vi "ME_acquire_5.vi"() -> ()   [LabVIEW 2015]
doc: "Use this template to build a producer/consumer design pattern. Use this template when you need to execute a process, such as data analysis, when a data source, such as a triggered acquisition, produces data at an uneven rate and you need to execute the process when the data becomes available."
uses:
  Mode.ctl
  oxford_driver/Oxford Drivers/BUSGEN.LLB/OxfordAddress.ctl
  <vilib>/Utility/file.llb/Write Delimited Spreadsheet (DBL).vi
  <vilib>/express/express arith-compare/Formula/XNode/ExpressFormulaBlockNode.xnode
  <vilib>/gmath/NI_Gmath.lvlib
panel:
  in  "stop 2":bool
  in  "dB":dbl=0.005
  in  "Dwell Time (ms)":u32=1
  out "appended array":dbl[][](array[numeric])
  in  "Magnet":bool
  out "Actual B Field (T)":dbl
  out "Actual Temperature (K)":dbl
  out "Actual Current (pA)":dbl
  in  "Sweep Field":bool
  in  "Tab Control":T1(tab)
  out "P(T)":cluster{dbl[], dbl[]}(graph)
  out "I(T)":cluster{dbl[], dbl[]}(graph)
  in  "Set temperature (K)":dbl=4.5
  in  "Temp Ramping Rate (K/min)":dbl=10.0
  in  "Heater Range":enum16{"Off", "Low", "Medium", "High"}(ring)
  in  "Heater On/Off":bool
  out "I(B) /Averaged/":cluster{"B array":dbl[], dbl[]}[](graph)
  out "I(B) 3":cluster{dbl[], dbl[]}[](graph)
  in  "Go to Set":bool
  in  "Set Field (T)":dbl=0.3
  in  "Field To Zero":bool
  in  "Sweep Rate (T/min)":dbl=2.0 format="%.6f"
  in  "Min Field (T)":dbl
  in  "Max Field (T)":dbl
  out "Up/Down":bool
  in  "Measure Noise":bool
  in  "Cycles":i32
  in  "maximum value":dbl=10.0 format="%0.2f"
  in  "minimum value":dbl=-10.0 format="%0.2f"
  in  "physical channels":tag="Dev1/ai1"
  out "PSD (pA/Hz^1/2) Peaks Removed":cluster{"f0":dbl, "df":dbl, "magnitude":dbl[]}(graph)
  out "PSD (pA/Hz^1/2)":cluster{"f0":dbl, "df":dbl, "magnitude":dbl[]}(graph)
  out "Current (pA) Filtered":waveform(dbl)(graph)
  out "Current (pA)":dbl[](graph)
  in  "Samples per channel":i32=1000
  in  "Rate":dbl=1000.0 format="%0.2f"
  in  "Cut-Off Frequency":dbl=100.0 caption="Lower Cut-Off"
  in  "Filter On":bool
  in  "Calibrate":bool
  in  "IV converter":refnum<visa-resource-name>="GPIB0::20::INSTR"
  in  "Magnetic Field":refnum<visa-resource-name>="GPIB0::21::INSTR"
  out "Time Lag":dbl=0.0500025749206543
  in  "Lake Shore":refnum<visa-resource-name>="GPIB0::11::INSTR"
  in  "Temp Refresh (s)":dbl=1.0
  in  "Sampling rate (Hz)":dbl=10.0
  in  "Gain (V/A)":dbl=1000000000.0
  in  "Sample area (mm^2)":dbl=3.9
  out "B_V":cluster{dbl[], "Best Linear Fit":dbl[]}[](graph)=[{[-0.00854253601, 0.00626134724, 0.0219834428, 0.0379117736, 0.0535871506, 0.0694316728, 0.0851615152, 0.100816481, 0.116478038, 0.132148461, 0.147876163, 0.16341701, 0.178976744, 0.194563632, 0.210251739, 0.225738944, 0.241298253, 0.256806034, 0.272344374, 0.287933477, 0.303494709, 0.318997125, 0.334591297, 0.350146681, 0.365618053, 0.380940961, 0.39666457, 0.412213675, 0.427724671, 0.443221444, 0.458760641, 0.474360042, 0.489915118, 0.505330598, 0.520967119, 0.536347531, 0.551813711, 0.567441155, 0.582995861, 0.598507522, 0.614041988, 0.629563151, 0.645106262, 0.660611914, 0.676136149, 0.691553948, 0.7071244, 0.72262999, 0.738171137, 0.753700392, 0.76919513, 0.784778028, 0.800215944, 0.8156961, 0.831325434, 0.846852183, 0.862326812, 0.877819169, 0.893312568, 0.90888536, 0.924354789], "Best Linear Fit"=[0.0, 0.005, 0.01, 0.015, 0.02, 0.025, 0.03, 0.035, 0.04, 0.045, 0.05, 0.055, 0.06, 0.065, 0.07, 0.075, 0.08, 0.085, 0.09, 0.095, 0.1, 0.105, 0.11, 0.115, 0.12, 0.125, 0.13, 0.135, 0.14, 0.145, 0.15, 0.155, 0.16, 0.165, 0.17, 0.175, 0.18, 0.185, 0.19, 0.195, 0.2, 0.205, 0.21, 0.215, 0.22, 0.225, 0.23, 0.235, 0.24, 0.245, 0.25, 0.255, 0.26, 0.265, 0.27, 0.275, 0.28, 0.285, 0.29, 0.295, 0.3]}, {[-0.00854253601, 0.00626134724, 0.0219834428, 0.0379117736, 0.0535871506, 0.0694316728, 0.0851615152, 0.100816481, 0.116478038, 0.132148461, 0.147876163, 0.16341701, 0.178976744, 0.194563632, 0.210251739, 0.225738944, 0.241298253, 0.256806034, 0.272344374, 0.287933477, 0.303494709, 0.318997125, 0.334591297, 0.350146681, 0.365618053, 0.380940961, 0.39666457, 0.412213675, 0.427724671, 0.443221444, 0.458760641, 0.474360042, 0.489915118, 0.505330598, 0.520967119, 0.536347531, 0.551813711, 0.567441155, 0.582995861, 0.598507522, 0.614041988, 0.629563151, 0.645106262, 0.660611914, 0.676136149, 0.691553948, 0.7071244, 0.72262999, 0.738171137, 0.753700392, 0.76919513, 0.784778028, 0.800215944, 0.8156961, 0.831325434, 0.846852183, 0.862326812, 0.877819169, 0.893312568, 0.90888536, 0.924354789], "Best Linear Fit"=[-0.00022554388023060128, 0.004536267537808887, 0.009593430775915074, 0.014716931562355689, 0.01975906732634002, 0.024855610270593523, 0.029915265354287977, 0.03495083565949541, 0.03998852608757118, 0.045029068349812316, 0.05008803495326229, 0.055086897848955874, 0.060091835929837946, 0.06510550835596321, 0.07015173884687344, 0.07513334727738563, 0.08013814865293042, 0.08512637555172443, 0.0901244320467579, 0.09513881694893507, 0.10014423687592358, 0.10513073807087174, 0.11014675346564809, 0.1151502923271957, 0.12012680792099008, 0.1250555686413888, 0.1301132186920259, 0.13511473785283767, 0.14010399888730068, 0.14508868495702945, 0.1500870171143548, 0.15510471446726903, 0.16010815425765457, 0.16506669165212906, 0.17009632901003072, 0.1750435864450521, 0.18001843198211442, 0.1850451496356715, 0.19004847041199868, 0.1950379453501071, 0.20003475573578386, 0.20502728708357412, 0.21002687821664084, 0.21501442030211, 0.220007939788244, 0.2249672231113706, 0.22997560874002893, 0.23496313088260184, 0.23996209027618054, 0.24495722449359253, 0.24994125598600042, 0.2549536449902534, 0.25991939913989753, 0.2648987401917687, 0.26992606578200207, 0.2749203939204135, 0.2798979571595809, 0.2848812227804405, 0.2898648235706211, 0.2948739618827834, 0.2998498524919418]}]
  out "V_I":cluster{dbl[], "Best Linear Fit":dbl[]}[](graph)=[{[0.0, 0.035, 0.069, 0.104, 0.138, 0.173, 0.208, 0.242, 0.277, 0.311, 0.346, 0.38, 0.415, 0.45, 0.484, 0.519, 0.553, 0.588, 0.623, 0.657, 0.692, 0.726, 0.761, 0.796, 0.83, 0.865, 0.899, 0.934, 0.969, 1.003, 1.038, 1.072, 1.107, 1.141, 1.176, 1.211, 1.245, 1.28, 1.314, 1.349, 1.384, 1.418, 1.453, 1.487, 1.522, 1.557, 1.591, 1.626, 1.66, 1.695, 1.73, 1.764, 1.799, 1.833, 1.868, 1.902, 1.937, 1.972, 2.006, 2.041, 2.075], "Best Linear Fit"=[-0.00854253601, 0.00626134724, 0.0219834428, 0.0379117736, 0.0535871506, 0.0694316728, 0.0851615152, 0.100816481, 0.116478038, 0.132148461, 0.147876163, 0.16341701, 0.178976744, 0.194563632, 0.210251739, 0.225738944, 0.241298253, 0.256806034, 0.272344374, 0.287933477, 0.303494709, 0.318997125, 0.334591297, 0.350146681, 0.365618053, 0.380940961, 0.39666457, 0.412213675, 0.427724671, 0.443221444, 0.458760641, 0.474360042, 0.489915118, 0.505330598, 0.520967119, 0.536347531, 0.551813711, 0.567441155, 0.582995861, 0.598507522, 0.614041988, 0.629563151, 0.645106262, 0.660611914, 0.676136149, 0.691553948, 0.7071244, 0.72262999, 0.738171137, 0.753700392, 0.76919513, 0.784778028, 0.800215944, 0.8156961, 0.831325434, 0.846852183, 0.862326812, 0.877819169, 0.893312568, 0.90888536, 0.924354789]}, {[0.0, 0.035, 0.069, 0.104, 0.138, 0.173, 0.208, 0.242, 0.277, 0.311, 0.346, 0.38, 0.415, 0.45, 0.484, 0.519, 0.553, 0.588, 0.623, 0.657, 0.692, 0.726, 0.761, 0.796, 0.83, 0.865, 0.899, 0.934, 0.969, 1.003, 1.038, 1.072, 1.107, 1.141, 1.176, 1.211, 1.245, 1.28, 1.314, 1.349, 1.384, 1.418, 1.453, 1.487, 1.522, 1.557, 1.591, 1.626, 1.66, 1.695, 1.73, 1.764, 1.799, 1.833, 1.868, 1.902, 1.937, 1.972, 2.006, 2.041, 2.075], "Best Linear Fit"=[-0.007846580254753975, 0.007882153481927697, 0.02316149482613275, 0.03889022856281441, 0.054169569907019474, 0.06989830364370113, 0.08562703738038281, 0.10090637872458785, 0.11663511246126955, 0.1319144538054746, 0.14764318754215625, 0.1629225288863613, 0.17865126262304296, 0.19437999635972467, 0.2096593377039297, 0.22538807144061138, 0.24066741278481643, 0.25639614652149806, 0.27212488025817977, 0.2874042216023848, 0.3031329553390665, 0.31841229668327153, 0.3341410304199532, 0.3498697641566349, 0.3651491055008399, 0.3808778392375216, 0.39615718058172666, 0.4118859143184083, 0.42761464805509, 0.442893989399295, 0.45862272313597674, 0.4739020644801818, 0.48963079821686345, 0.5049101395610684, 0.5206388732977502, 0.5363676070344319, 0.5516469483786369, 0.5673756821153185, 0.5826550234595236, 0.5983837571962053, 0.6141124909328869, 0.629391832277092, 0.6451205660137737, 0.6603999073579787, 0.6761286410946604, 0.691857374831342, 0.7071367161755471, 0.7228654499122288, 0.7381447912564338, 0.7538735249931156, 0.7696022587297972, 0.7848816000740022, 0.8006103338106839, 0.815889675154889, 0.8316184088915707, 0.8468977502357756, 0.8626264839724573, 0.878355217709139, 0.893634559053344, 0.9093632927900257, 0.9246426341342309]}]
  out "B0 (T)":dbl=0.0025222449819540214
  out "B/V (T/V)":dbl=0.321659617116981
  out "I0 (A)":dbl=-0.007846580254753975
  out "V/I (Ohm)":dbl=0.44939239247661916
  in  "dt (s)":dbl=0.05
  in  "Temp/Magnetic Field":bool
  out "Save":dbl[][](array[numeric])
  out "output array":dbl[][](array[numeric])
  out "index":i8
  out "Read?":bool
  out "Magnetic Field (T)":dbl[](array[numeric])
  out "Reset":bool
  out "Measured Current (pA)":dbl[](array[numeric])
  out "Elapsed Time (s)":dbl[](array[numeric])
  out "Start time":timestamp
  in  "Enum":T2
  out "B array":dbl[](array[numeric])
  in  "dB (T)":dbl=0.0001
  in  "Counter":i8
  out "L magnet (H)":dbl
  out "R magnet (mOhm)":dbl
  out "Actual Current (R0)":dbl
  out "Actual Field (T)":dbl
  out "Temperature array":dbl[](array[numeric])
  in  "New Measurement File":bool
  out "Measurement File":path
  out "refnum out":refnum<file>
  in  "Measuring":bool
  in  "Measure (Start/Pause)":bool
  in  "stop":bool
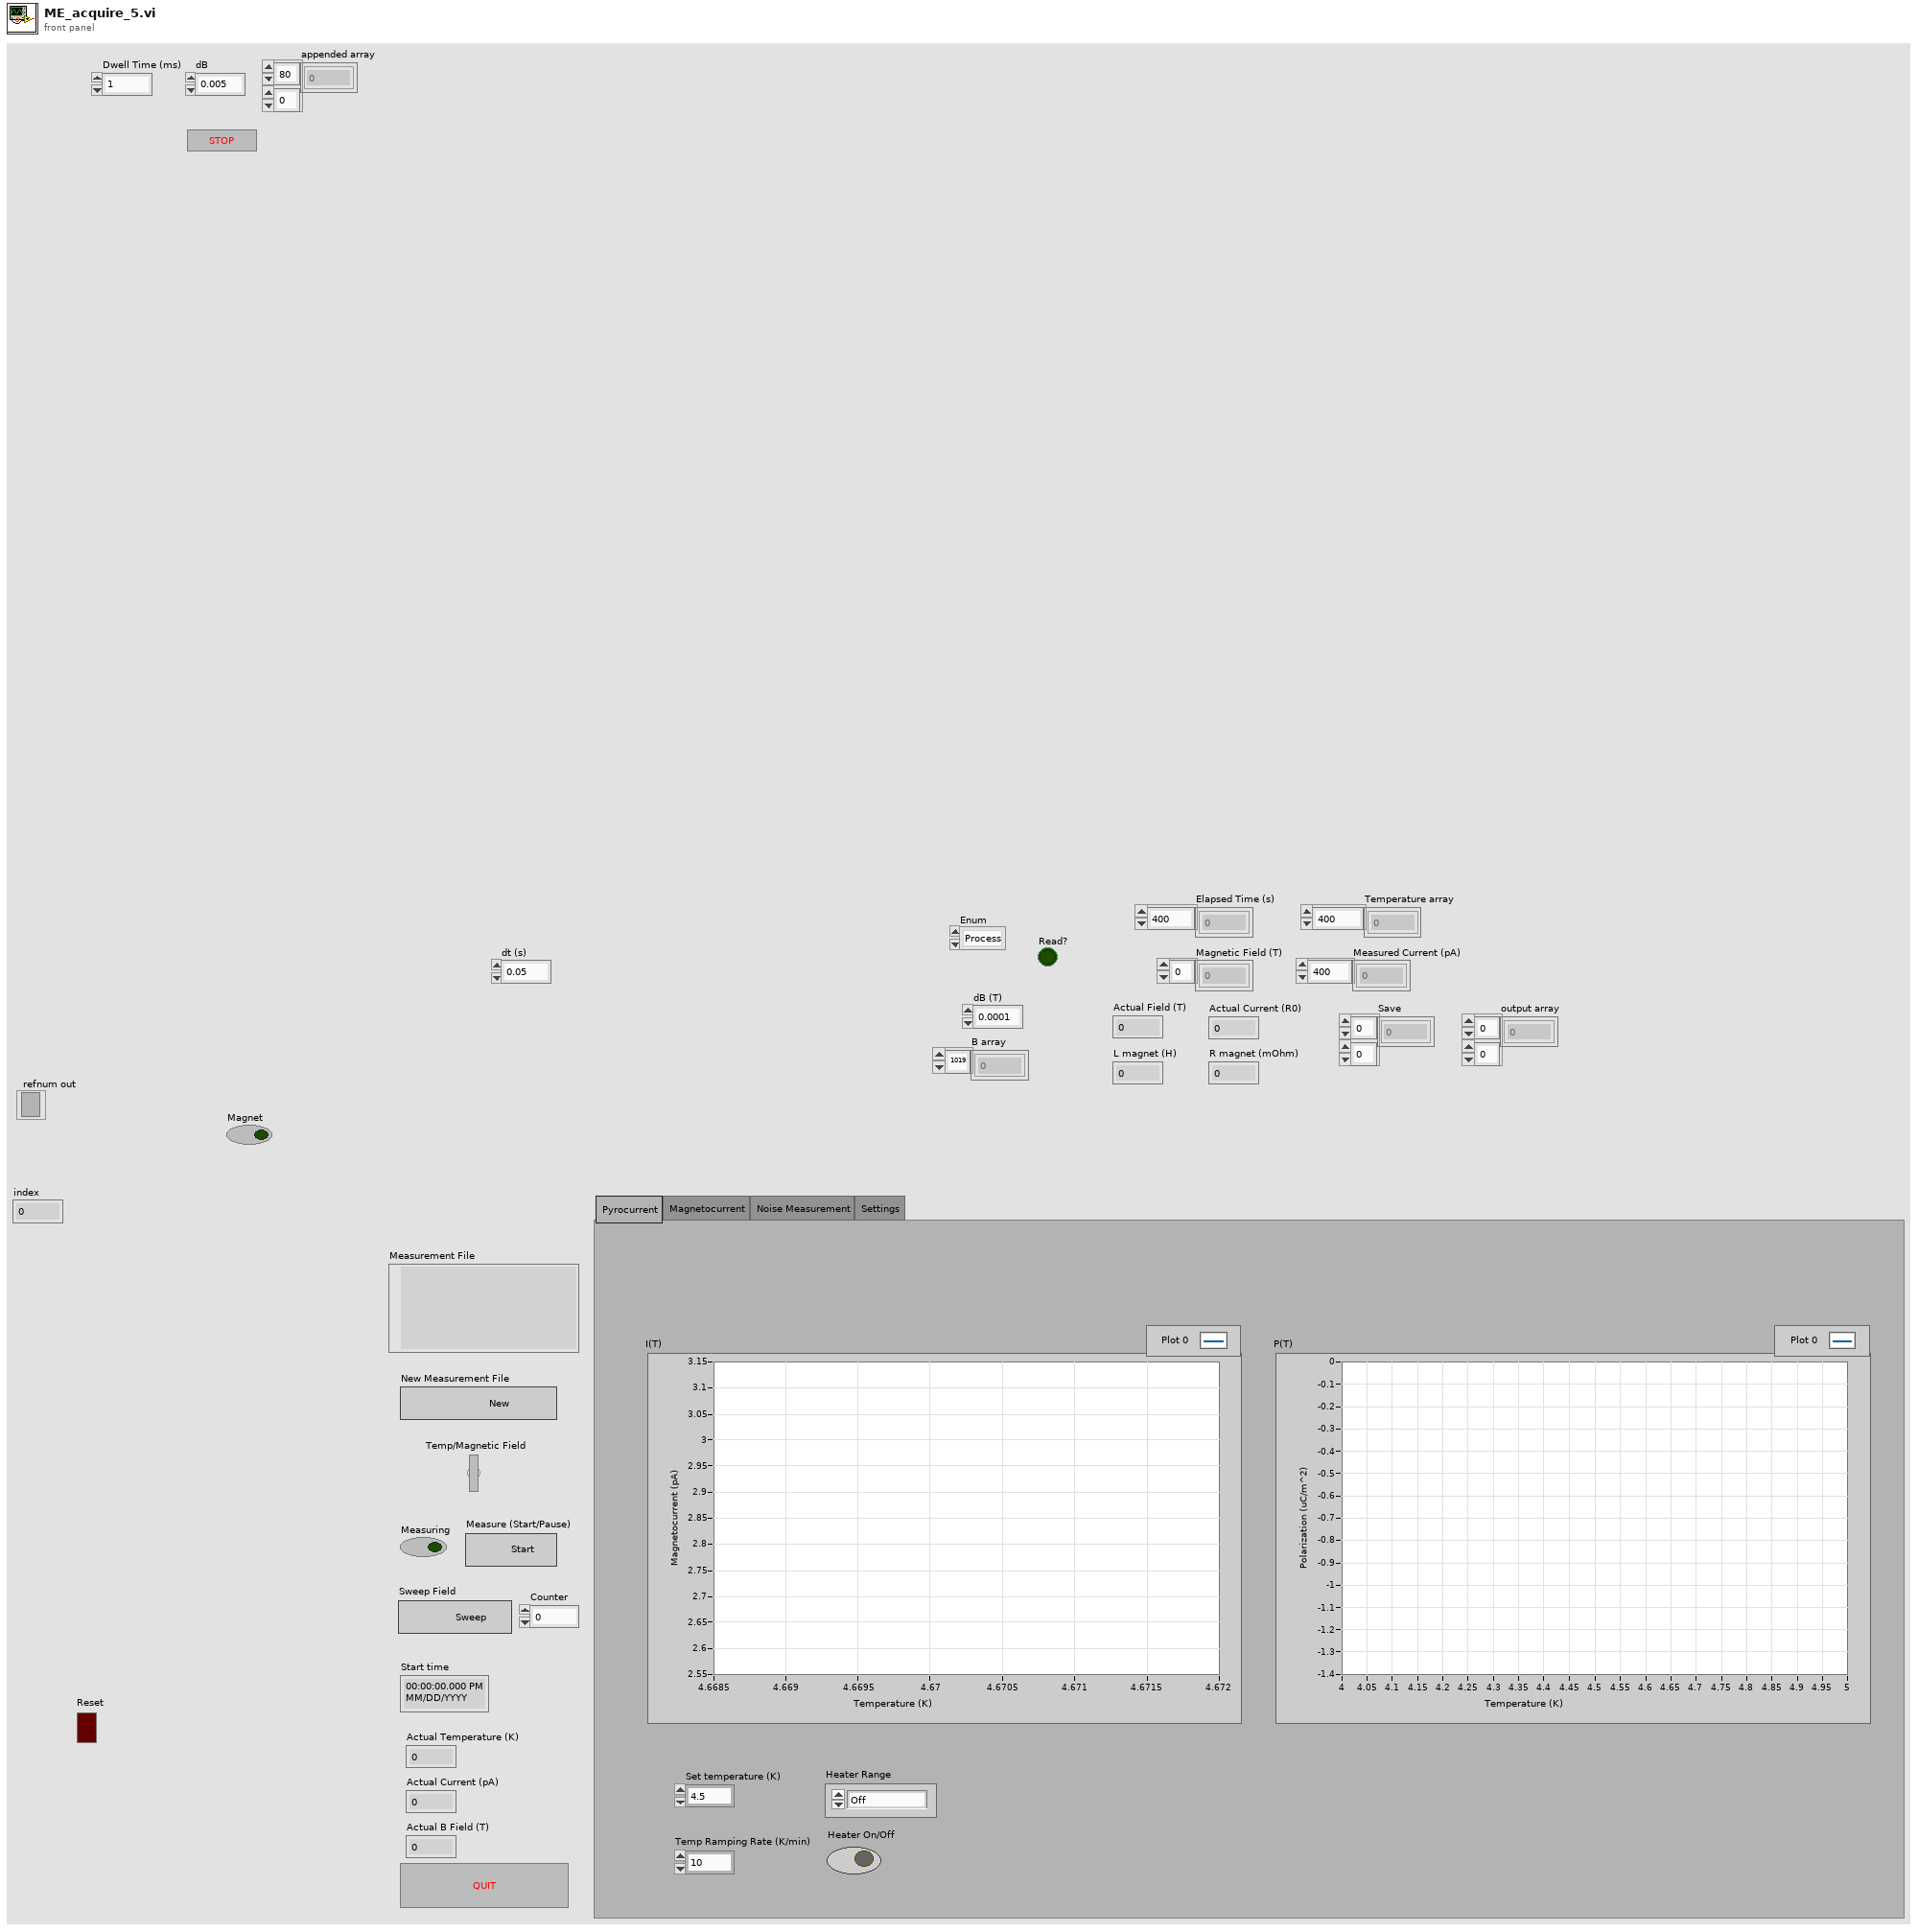
[diagram p1: front panel]
types:
  T1 = enum32{"Pyrocurrent", "Magnetocurrent", "Noise Measurement", "Settings"}
  T2 = typedef "Mode.ctl" = enum16{"Process", "Plot", "Save", "Return"}
  T3 = enum16{"open", "replace", "create", "open or create", "replace or create", "replace or create with confirmation"}
  T4 = typedef "OxfordAddress.ctl" = cluster{"Com Port":i32, "ISOBUS Address":i32, "GPIB Address":i16, "Communication":enum16{"RS232", "ISOBUS", "GPIB", "Gateway"}}
  T5 = cluster{"seconds since 1Jan1904":timestamp, "read buffer":string, "read buffer":string}
  T6 = cluster{"I array out (A)":dbl[], "V array out (V)":dbl[]}
  T7 = cluster{"I array out (A)":dbl[], "Best Linear Fit":dbl[]}
  T8 = cluster{"V array out (V)":dbl[], "B array Out":dbl[]}
  T9 = cluster{"V array out (V)":dbl[], "Best Linear Fit 2":dbl[]}
  T10 = cluster{"I array out (A)":dbl[], "Best Linear Fit":dbl[]}[]
  T11 = cluster{"V array out (V)":dbl[], "Best Linear Fit 2":dbl[]}[]
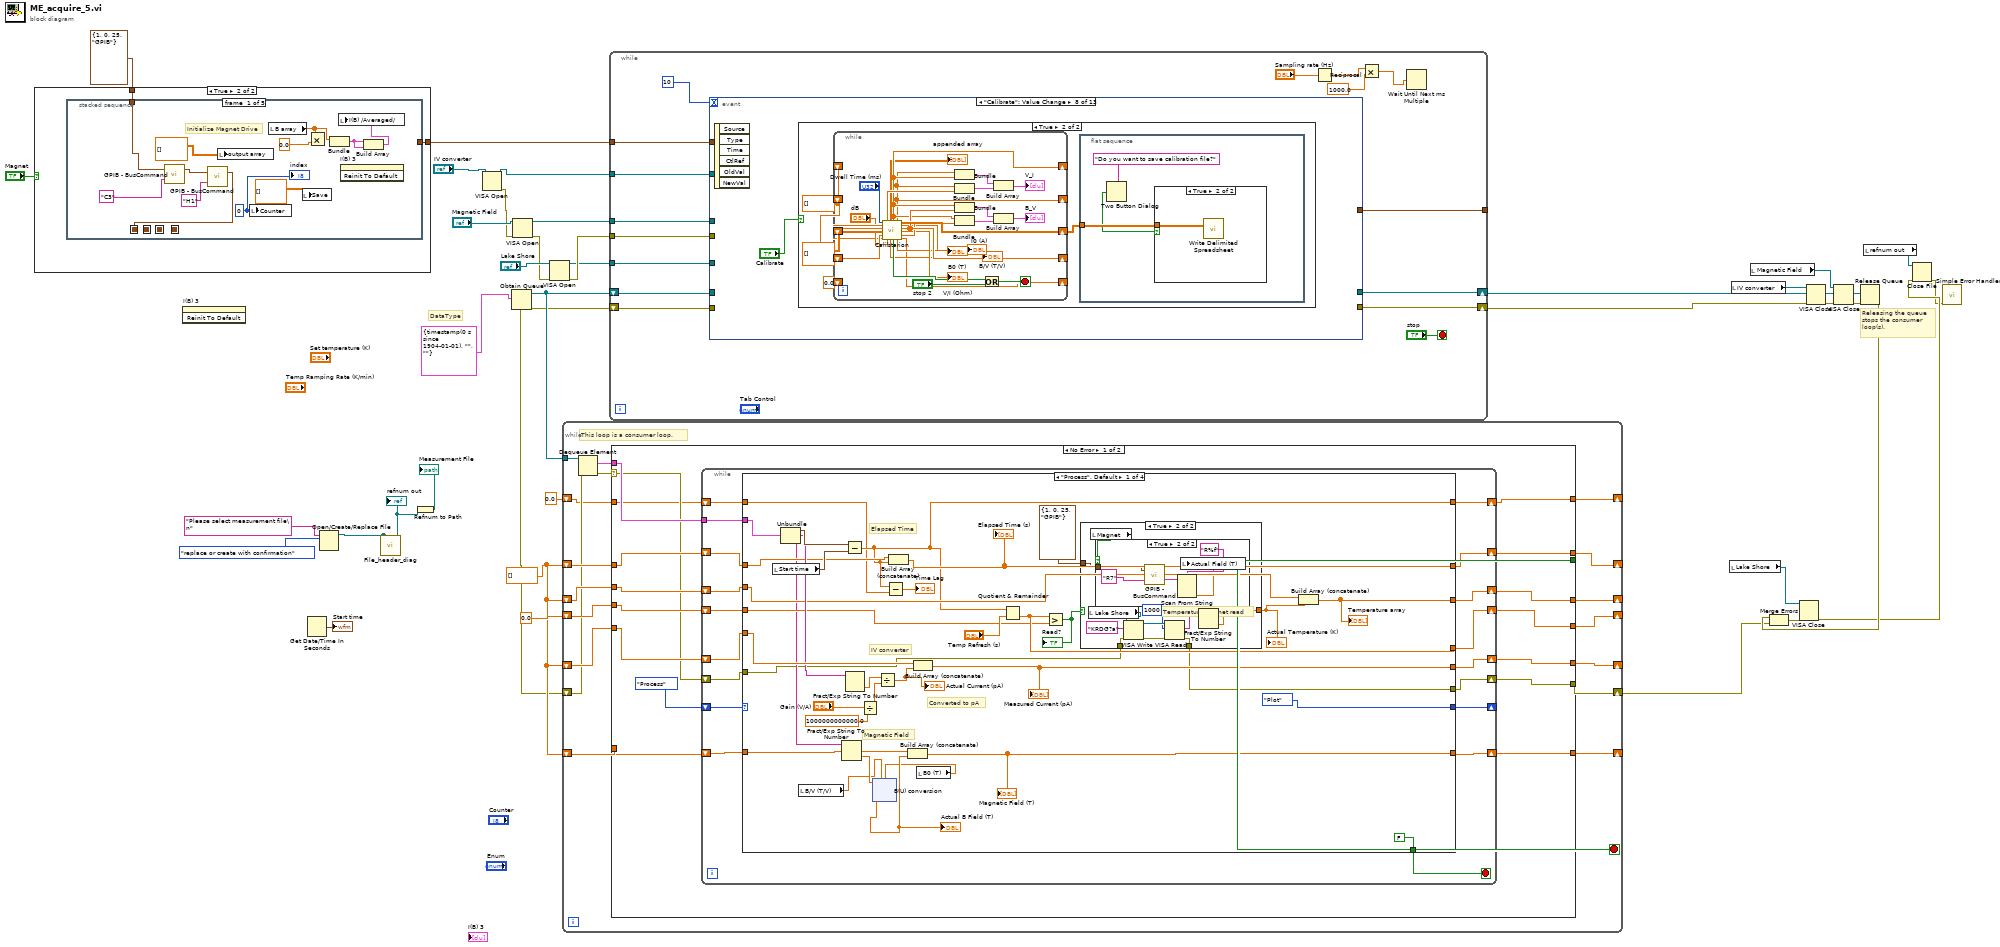
[diagram p0: block diagram]
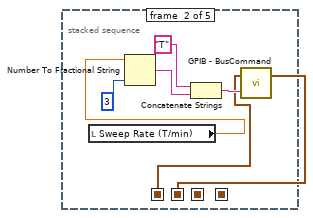
[diagram p3: hidden frame]
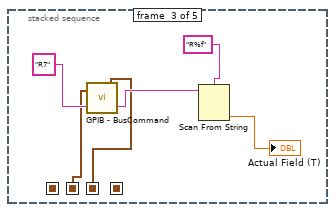
[diagram p4: hidden frame]
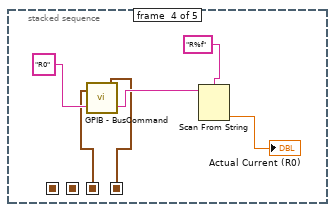
[diagram p5: hidden frame]
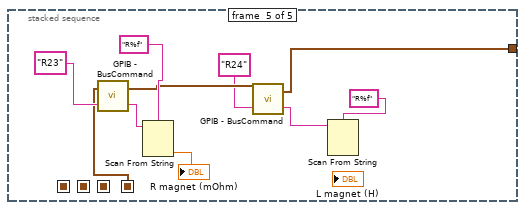
[diagram p6: hidden frame]
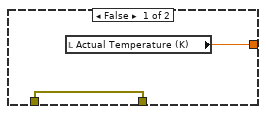
[diagram p7: hidden frame]
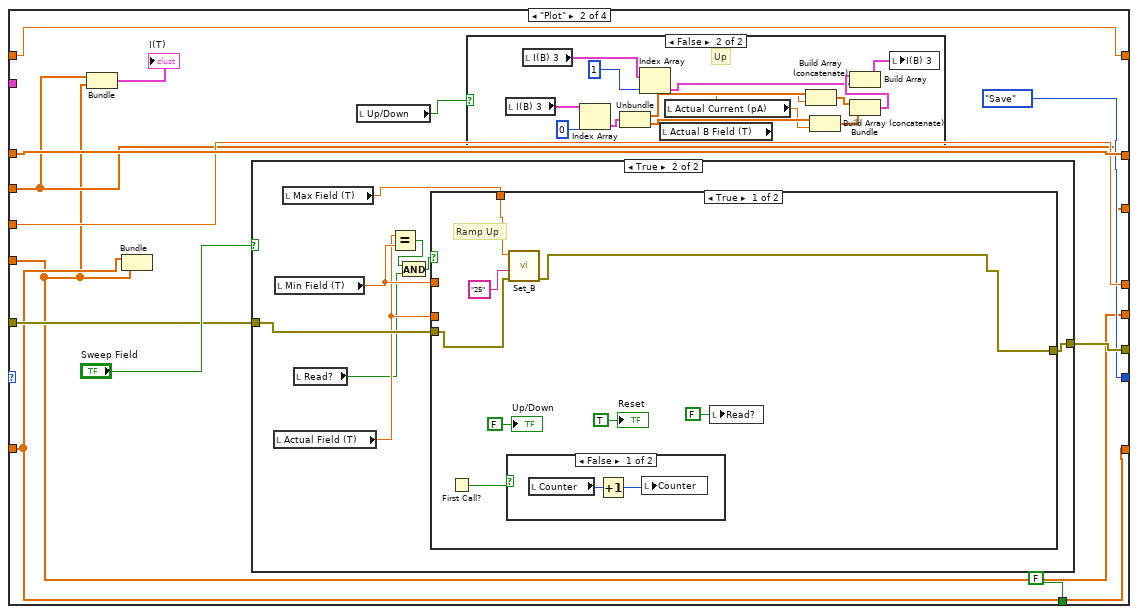
[diagram p9: hidden frame]
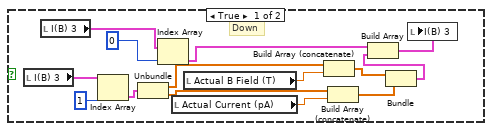
[diagram p10: hidden frame]
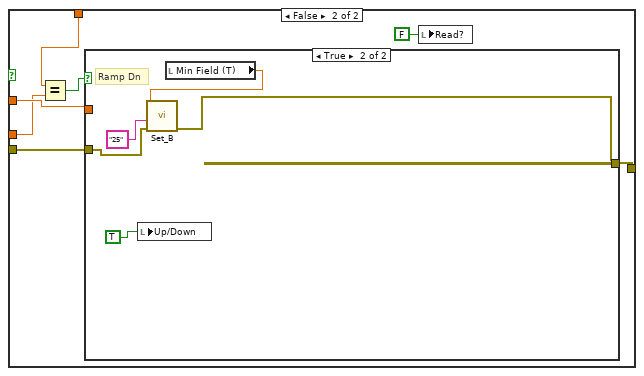
[diagram p13: hidden frame]
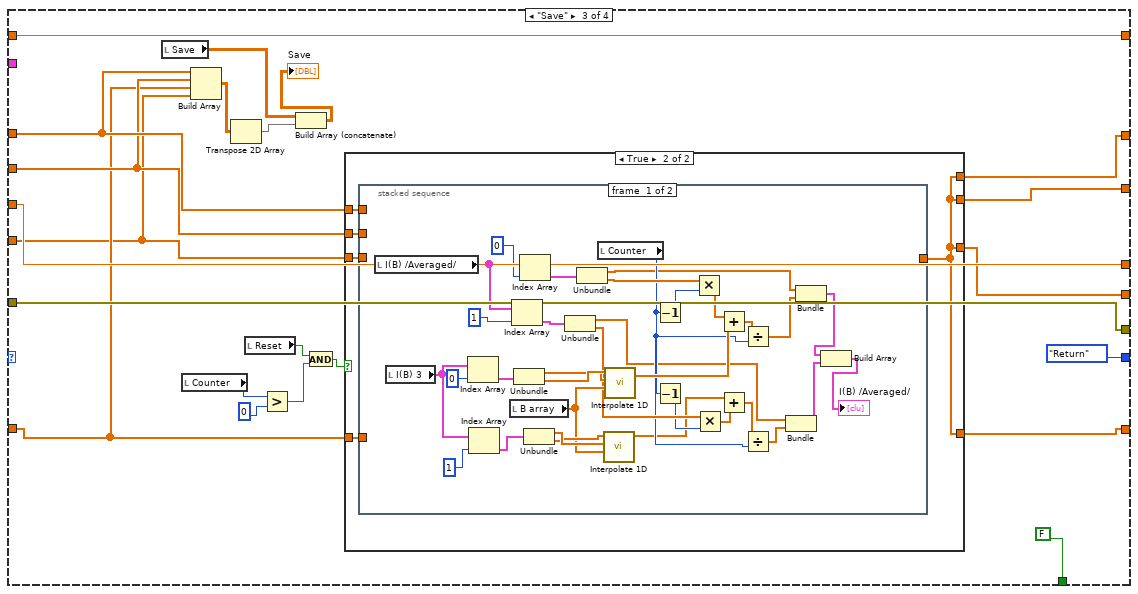
[diagram p15: hidden frame]
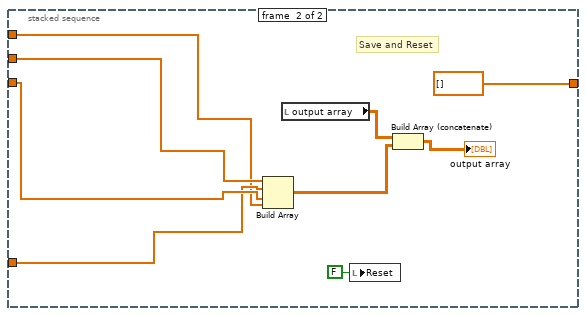
[diagram p17: hidden frame]
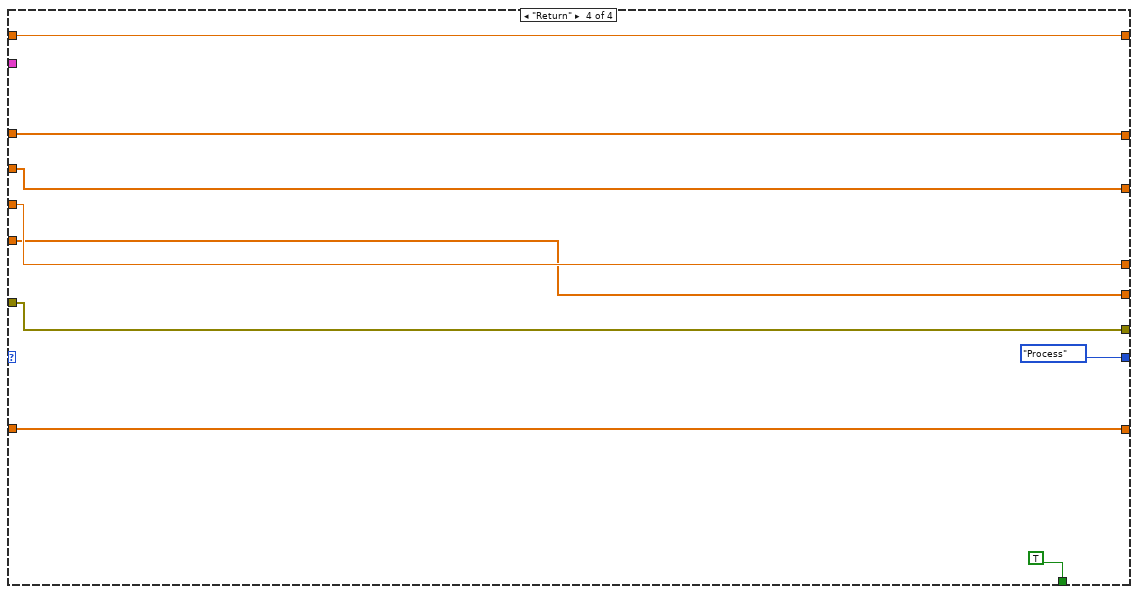
[diagram p18: hidden frame]
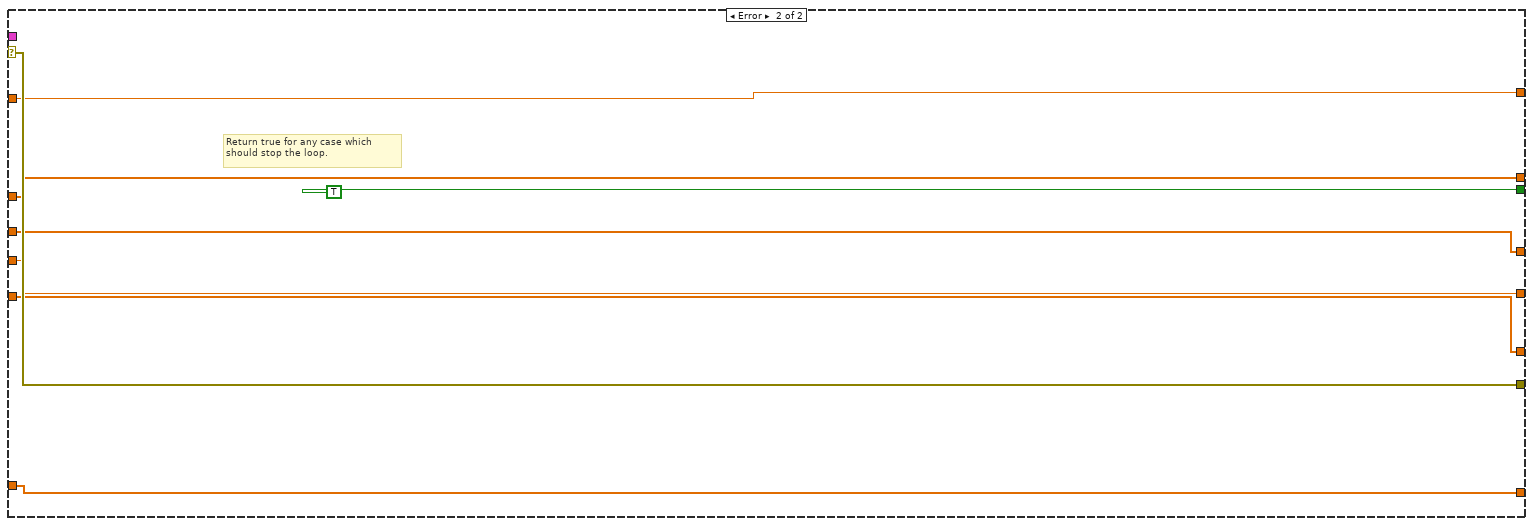
[diagram p19: hidden frame]
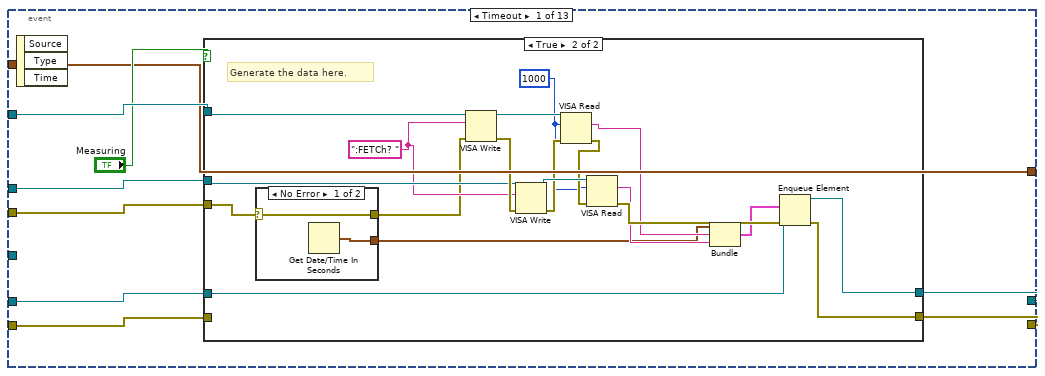
[diagram p20: hidden frame]
diagram:
  w6 = dbl[] []
  # "DataType"
  # "Releasing the queue stops the consumer loop(s)."
  n1 = case shown="True" "Magnet" {
    tunnel: T4 {"Com Port"=1, "ISOBUS Address"=0, "GPIB Address"=25, "Communication"=enum."GPIB"} ("Address") -> [w37 w39]
    tunnel: [w37 w38] -> w15
    frame False {
    }
    frame True {
      n2 = stacked-sequence {
        seq-local: [w49 _ _ _ _] -> [_ w54 _ _ _]
        seq-local: [_ w53 _ _ _] -> [_ _ w61 _ _]
        seq-local: [_ _ w60 _ _] -> [_ _ _ w67 _]
        seq-local: [_ _ _ w66 _] -> [_ _ _ _ w77]
        tunnel: w39 -> [w51 _ _ _ _]
        tunnel: [_ _ _ _ w75] -> w38
        frame #0 {
          w47 = i8 0 ("Counter")
          # "Initialize Magnet Drive"
          n3 = call "GPIB - BusCommand.vi"("Command"="C3", "Address"=w51) -> ("Address(thru)"=w50:T4)  [unwired: 1 out]
          n4 = call "GPIB - BusCommand.vi"("Command"="H1", "Address"=w50) -> ("Address(thru)"=w49:T4)  [unwired: 1 out]
          n5 = local write "output array"(dbl[][] []) -> ()
          n6 = local write "Counter"(w47) -> ()
          n7 = local read "B array"() -> (w45:dbl[])
          n8 = local write "Save"(dbl[][] [] ("Save")) -> ()
          n9 = Multiply(x=w45, y=0.0) -> (x*y=w44:dbl[])
          n10 = Bundle("B array"=w45, w44) -> (w43:cluster{"B array":dbl[], dbl[]})  [unwired: 1 in]
          n11 = invoke on="I(B) 3" class="XYGraph (strict)" method="Reinit To Default"() -> ()  [unwired: 3 in, 3 out]
          n12 = Build Array(w43, w43) -> (w42:cluster{"B array":dbl[], dbl[]}[])
          n13 = local write "I(B) /Averaged/"(w42) -> ()
          "index" <- w47
        }
        frame #1 {
          n14 = local read "Sweep Rate (T/min)"() -> (w55:dbl)
          n15 = Number To Fractional String(number=w55, precision (6)=i16 3) -> (F-format string=w57:string)  [unwired: 2 in]
          n16 = Concatenate Strings("T" ("format string"), w57) -> (w56:string)
          n17 = call "GPIB - BusCommand.vi"("Command"=w56, "Address"=w54) -> ("Address(thru)"=w53:T4)  [unwired: 1 out]
        }
        frame #2 {
          n18 = call "GPIB - BusCommand.vi"("Command"="R7" ("format string"), "Address"=w61) -> ("Reply"=w65:string, "Address(thru)"=w60:T4)
          n19 = Scan From String(format string="R%f" ("remaining string"), input string=w65) -> (output 1=→"Actual Field (T)":dbl)  [unwired: 3 in, 3 out]
        }
        frame #3 {
          n20 = call "GPIB - BusCommand.vi"("Command"="R0" ("format string"), "Address"=w67) -> ("Reply"=w71:string, "Address(thru)"=w66:T4)
          n21 = Scan From String(format string="R%f" ("remaining string"), input string=w71) -> (output 1=→"Actual Current (R0)":dbl)  [unwired: 3 in, 3 out]
        }
        frame #4 {
          n22 = call "GPIB - BusCommand.vi"("Command"="R23" ("format string"), "Address"=w77) -> ("Reply"=w81:string, "Address(thru)"=w76:T4)
          n23 = Scan From String(format string="R%f" ("remaining string"), input string=w81) -> (output 1=→"R magnet (mOhm)":dbl)  [unwired: 3 in, 3 out]
          n24 = call "GPIB - BusCommand.vi"("Command"="R24" ("format string"), "Address"=w76) -> ("Reply"=w73:string, "Address(thru)"=w75:T4)
          n25 = Scan From String(format string="R%f" ("remaining string"), input string=w73) -> ()  [unwired: 4 in, 3 out]
        }
      }
    }
  }
  n26 = invoke on="I(B) 3" class="XYGraph (strict)" method="Reinit To Default"() -> ()  [unwired: 3 in, 3 out]
  n27 = Get Date/Time In Seconds() -> (seconds since 1Jan1904=→"Start time":timestamp)
  n28 = Open/Create/Replace File(prompt="Please select measurement file\n", operation (0:open)=T3."replace or create with confirmation") -> (refnum out=w11:refnum<file>)  [unwired: 4 in, 2 out]
  "refnum out" <- w11
  n29 = call "File_header_diag.vi"("Byte Stream File in"=w11) -> ()  [unwired: 11 in]
  n30 = Refnum to Path(1:w11) -> (0:→"Measurement File":path)
  n31 = VISA Open(VISA resource name="IV converter") -> (VISA resource name=w31:refnum<visa-resource-name>, error out=w33:errorcluster)  [unwired: 4 in]
  n32 = Obtain Queue(element data type=T5 {"seconds since 1Jan1904"=timestamp(0 s since 1904-01-01), "read buffer"="", "read buffer"=""} ("output cluster")) -> (queue out=w36:refnum<queue>, error out=w4:errorcluster)  [unwired: 4 in, 1 out]
  n33 = VISA Open(error in (no error)=w33, VISA resource name="Magnetic Field") -> (VISA resource name=w30:refnum<visa-resource-name>, error out=w8:errorcluster)  [unwired: 3 in]
  n34 = VISA Open(error in (no error)=w8, VISA resource name="Lake Shore") -> (VISA resource name=w2:refnum<visa-resource-name>, error out=w7:errorcluster)  [unwired: 3 in]
  n35 = while {
    tunnel: w36 -> [w99]
    shift-right: [w94] -> _
    shift-left: w6 -> [w93]
    shift-right: [w92] -> _
    shift-left: w6 -> [w91]
    shift-right: [w90] -> _
    shift-left: w6 -> [w89]
    shift-right: [w88] -> _
    shift-left: 0.0 -> [w87]
    shift-right: [w86] -> _
    shift-left: w6 -> [w85]
    shift-right: [w95] -> w20
    shift-left: w4 -> [w84]
    shift-right: [w83] -> _
    shift-left: 0.0 -> [w82]
    stop <- w96 stop-if-true
    # "This loop is a consumer loop."
    n36 = Dequeue Element(queue=w99, error in (no error)=w84) -> (element=w97:T5, error out=w98:errorcluster)  [unwired: 1 in, 2 out]
    n37 = case shown="No Error" w98 {
      selector: w98 -> [w103 w360]
      tunnel: w97 -> [w114 _]
      tunnel: [_ TRUE] -> w96
      tunnel: [w102 w360] -> w95
      tunnel: [w113 w359] -> w94
      tunnel: w93 -> [w112 w359]
      tunnel: [w111 w356] -> w92
      tunnel: w91 -> [w110 w356]
      tunnel: [w109 w355] -> w90
      tunnel: w89 -> [w108 w355]
      tunnel: [w107 w357] -> w88
      tunnel: w87 -> [w106 w357]
      tunnel: [w105 w358] -> w86
      tunnel: w85 -> [w104 w358]
      tunnel: [w101 w354] -> w83
      tunnel: w82 -> [w100 w354]
      frame No Error {
        n38 = while {
          shift-right: [w121] -> _
          shift-left: Mode."Process" ("Enum") -> [w133]
          tunnel: w114 -> [w132]
          shift-right: [w131] -> w113
          shift-left: w112 -> [w130]
          shift-right: [w123] -> w105
          shift-left: w104 -> [w122]
          shift-right: [w125] -> w107
          shift-left: w106 -> [w124]
          shift-right: [w129] -> w111
          shift-left: w110 -> [w128]
          shift-right: [w119] -> w102
          shift-left: w103 -> [w120]
          shift-right: [w127] -> w109
          shift-left: w108 -> [w126]
          shift-right: [w117] -> w101
          shift-left: w100 -> [w116]
          stop <- w118 stop-if-true
          n39 = case shown="\"Process\", Default" w133 {
            tunnel: w132 -> [w166 _ _ _]
            tunnel: [w163 w208 w280 w352] -> w131
            tunnel: w130 -> [w154 w208 w279 w352]
            tunnel: [w162 w200 w282 w349] -> w129
            tunnel: w128 -> [w161 w200 w276 w349]
            tunnel: [w158 w204 w283 w346] -> w127
            tunnel: w126 -> [w157 w204 w277 w346]
            tunnel: [w153 w207 w291 w350] -> w125
            tunnel: w124 -> [w152 w207 w291 w350]
            tunnel: [w149 w201 w281 w351] -> w123
            tunnel: w122 -> [w150 w201 w278 w351]
            tunnel: [Mode."Plot" ("Enum") Mode."Save" ("Enum") Mode."Return" ("Enum") Mode."Process" ("Enum")] -> w121
            tunnel: w120 -> [w145 w210 w290 w348]
            tunnel: [w144 w209 w290 w348] -> w119
            tunnel: [FALSE FALSE FALSE TRUE] -> w118
            tunnel: [w141 w203 w289 w345] -> w117
            tunnel: w116 -> [w140 w203 w289 w345]
            frame "Process", Default {
              # "Converted to pA"
              # "Magnetic Field"
              # "IV converter"
              # "Elapsed Time"
              n40 = local read "Start time"() -> (w164:timestamp)
              n41 = Unbundle(w166) -> ("seconds since 1Jan1904"=w165:timestamp, "read buffer"=w159:string, "read buffer"=w146:string)
              n42 = local read "B/V (T/V)"() -> (w135:dbl)
              n43 = Fract/Exp String To Number(string=w146) -> (number=w156:dbl)  [unwired: 3 in, 1 out]
              n44 = Subtract(x=w165, y=w164) -> (x-y=w141:dbl)
              n45 = Fract/Exp String To Number(string=w159) -> (number=w160:dbl)  [unwired: 3 in, 1 out]
              n46 = Divide(x="Gain (V/A)", y=1000000000000.0) -> (x/y=w138:dbl)
              n47 = Divide(x=w160, y=w138) -> (x/y=w139:dbl)
              "Actual Current (pA)" <- w139
              n48 = Subtract(x=w141, y=w140) -> (x-y=→"Time Lag":dbl)
              n49 = Build Array (concatenate)(w154, w141) -> (w163:dbl[])
              "Elapsed Time (s)" <- w163
              n50 = Build Array (concatenate)(w161, w139) -> (w162:dbl[])
              "Measured Current (pA)" <- w162
              n51 = local read "B0 (T)"() -> (w134:dbl)
              n52 = xnode "B(U) conversion"("V"=w156, "BpV"=w135, "B0"=w134) -> ("Result"=w155:dbl)  [unwired: 1 in, 1 out]
              "Actual B Field (T)" <- w155
              n53 = Build Array (concatenate)(w157, w155) -> (w158:dbl[])
              "Magnetic Field (T)" <- w158
              n54 = Quotient & Remainder(x=w141, y="Temp Refresh (s)") -> (floor(x/y)=w153:dbl)  [unwired: 1 out]
              n55 = Greater?(x=w153, y=w152) -> (0:w151:bool)
              "Read?" <- w151
              n56 = case shown="True" w151 {
                tunnel: [w170 w176] -> w148
                tunnel: w145 -> [w169 w175]
                tunnel: [w169 w174] -> w144
                tunnel: T4 {"Com Port"=1, "ISOBUS Address"=0, "GPIB Address"=25, "Communication"=enum."GPIB"} ("Address") -> [_ w173]
                frame False {
                  n57 = local read "Actual Temperature (K)"() -> (w170:dbl)
                }
                frame True {
                  # "Temperature/Magnet read"
                  n58 = local read "Lake Shore"() -> (w172:refnum<visa-resource-name>)
                  n59 = local read "Magnet"() -> (w171:bool)
                  n60 = case shown="True" w171 {
                    tunnel: w173 -> [_ w183]
                    frame False {
                    }
                    frame True {
                      n61 = call "GPIB - BusCommand.vi"("Command"="R7" ("format string"), "Address"=w183) -> ("Reply"=w184:string)  [unwired: 1 out]
                      n62 = Scan From String(format string="R%f" ("remaining string"), input string=w184) -> (output 1=w182:dbl)  [unwired: 3 in, 3 out]
                      n63 = local write "Actual Field (T)"(w182) -> ()
                    }
                  }
                  n64 = VISA Write(VISA resource name=w172, write buffer="KRDG?a", error in (no error)=w175) -> (VISA resource name out=w180:refnum<visa-resource-name>, error out=w179:errorcluster)  [unwired: 1 out]
                  n65 = VISA Read(VISA resource name=w180, byte count=u32 1000, error in (no error)=w179) -> (read buffer=w177:string, error out=w174:errorcluster)  [unwired: 2 out]
                  n66 = Fract/Exp String To Number(string=w177) -> (number=w176:dbl)  [unwired: 3 in, 1 out]
                }
              }
              "Actual Temperature (K)" <- w148
              n67 = Build Array (concatenate)(w150, w148) -> (w149:dbl[])
              "Temperature array" <- w149
            }
            frame "Plot" {
              n68 = Bundle(w201, w200) -> (→"I(T)":cluster{dbl[], dbl[]})  [unwired: 1 in]
              n69 = Bundle(w204, w200) -> ()  [unwired: 1 in, 1 out]
              n70 = case shown="True" "Sweep Field" {
                tunnel: [w240 w248] -> w209
                tunnel: w210 -> [w240 w245]
                frame False {
                }
                frame True {
                  n71 = local read "Actual Field (T)"() -> (w244:dbl)
                  n72 = local read "Min Field (T)"() -> (w246:dbl)
                  n73 = local read "Max Field (T)"() -> (w247:dbl)
                  n74 = local read "Read?"() -> (w241:bool)
                  n75 = Equal?(x=w244, y=w246) -> (x = y?=w243:bool)
                  n76 = And(x=w243, y=w241) -> (x .and. y?=w242:bool)
                  n77 = case shown="True" w242 {
                    tunnel: [w255 w265] -> w248
                    tunnel: w247 -> [w256 w264]
                    tunnel: w246 -> [_ w263]
                    tunnel: w244 -> [_ w261]
                    tunnel: w245 -> [w254 w260]
                    frame True {
                      # "Ramp Up"
                      n78 = First Call?() -> (First Call?: T/F=w249:bool)
                      n79 = case shown="False" w249 {
                        frame False {
                          n80 = local read "Counter"() -> (w257:i8)
                          n81 = Increment(x=w257) -> (x+1=w258:i8)
                          n82 = local write "Counter"(w258) -> ()
                        }
                        frame True {
                        }
                      }
                      n83 = call "Set_B.vi"("error in (no error)"=w254, "address string"="25", "Set Field (T)"=w256) -> ("error out"=w255:errorcluster)  [unwired: 8 in]
                      n84 = local write "Read?"(FALSE ("Read?")) -> ()
                      "Up/Down" <- FALSE ("Up/Down")
                      "Reset" <- TRUE ("Save")
                    }
                    frame False {
                      n85 = Equal?(x=w264, y=w261) -> (x = y?=w262:bool)
                      n86 = case shown="True" w262 {
                        tunnel: [w266 w268] -> w265
                        tunnel: w263 -> [_ _]
                        tunnel: w260 -> [w266 w269]
                        frame False {
                        }
                        frame True {
                          # "Ramp Dn"
                          n87 = local write "Up/Down"(TRUE ("Up/Down")) -> ()
                          n88 = local read "Min Field (T)"() -> (w267:dbl)
                          n89 = call "Set_B.vi"("error in (no error)"=w269, "address string"="25", "Set Field (T)"=w267) -> ("error out"=w268:errorcluster)  [unwired: 8 in]
                        }
                      }
                      n90 = local write "Read?"(FALSE ("Read?")) -> ()
                    }
                  }
                }
              }
              n91 = local read "Up/Down"() -> (w202:bool)
              n92 = case shown="False" w202 {
                frame True {
                  # "Down"
                  n93 = local read "I(B) 3"() -> (w221:cluster{dbl[], dbl[]}[])
                  n94 = local read "I(B) 3"() -> (w225:cluster{dbl[], dbl[]}[])
                  n95 = Index Array(array=w221, index=1) -> (element=w219:cluster{dbl[], dbl[]})
                  n96 = Unbundle(w219) -> (w218:dbl[], w217:dbl[])
                  n97 = Index Array(array=w225, index=i8 0 ("t")) -> (element=w222:cluster{dbl[], dbl[]})
                  n98 = local read "Actual Current (pA)"() -> (w214:dbl)
                  n99 = local read "Actual B Field (T)"() -> (w213:dbl)
                  n100 = Build Array (concatenate)(w218, w213) -> (w216:dbl[])
                  n101 = Build Array (concatenate)(w217, w214) -> (w215:dbl[])
                  n102 = Bundle(w216, w215) -> (w212:cluster{dbl[], dbl[]})  [unwired: 1 in]
                  n103 = Build Array(w222, w212) -> (w223:cluster{dbl[], dbl[]}[])
                  n104 = local write "I(B) 3"(w223) -> ()
                }
                frame False {
                  # "Up"
                  n105 = local read "I(B) 3"() -> (w237:cluster{dbl[], dbl[]}[])
                  n106 = local read "I(B) 3"() -> (w239:cluster{dbl[], dbl[]}[])
                  n107 = Index Array(array=w237, index=0) -> (element=w235:cluster{dbl[], dbl[]})
                  n108 = Unbundle(w235) -> (w234:dbl[], w233:dbl[])
                  n109 = Index Array(array=w239, index=i8 1 ("t")) -> (element=w227:cluster{dbl[], dbl[]})
                  n110 = local read "Actual B Field (T)"() -> (w229:dbl)
                  n111 = local read "Actual Current (pA)"() -> (w228:dbl)
                  n112 = Build Array (concatenate)(w234, w229) -> (w232:dbl[])
                  n113 = Build Array (concatenate)(w233, w228) -> (w231:dbl[])
                  n114 = Bundle(w232, w231) -> (w230:cluster{dbl[], dbl[]})  [unwired: 1 in]
                  n115 = Build Array(w230, w227) -> (w226:cluster{dbl[], dbl[]}[])
                  n116 = local write "I(B) 3"(w226) -> ()
                }
              }
            }
            frame "Save" {
              n117 = local read "Save"() -> (w272:dbl[][])
              n118 = local read "Counter"() -> (w288:i8)
              n119 = Build Array(w279, w278, w277, w276) -> (w275:dbl[][])
              n120 = Transpose 2D Array(2D array=w275) -> (transposed array=w274:dbl[][])
              n121 = local read "Reset"() -> (w285:bool)
              n122 = Greater?(x=w288, y=i8 0) -> (0:w284:bool)
              n123 = Build Array (concatenate)(w272, w274) -> (→"Save":dbl[][])
              n124 = And(x=w285, y=w284) -> (x .and. y?=w286:bool)
              n125 = case shown="True" w286 {
                tunnel: w277 -> [w297 w298]
                tunnel: [w297 w302] -> w283
                tunnel: w276 -> [w296 w299]
                tunnel: [w296 w302] -> w282
                tunnel: w278 -> [w295 w300]
                tunnel: [w295 w302] -> w281
                tunnel: w279 -> [w294 w301]
                tunnel: [w294 w302] -> w280
                frame False {
                }
                frame True {
                  n126 = stacked-sequence {
                    tunnel: [_ dbl[] []] -> w302
                    tunnel: w301 -> [_ w337]
                    tunnel: w300 -> [_ w342]
                    tunnel: w299 -> [_ w339]
                    tunnel: w298 -> [_ w338]
                    frame #0 {
                      n127 = local read "I(B) /Averaged/"() -> (w325:cluster{"B array":dbl[], dbl[]}[])
                      n128 = local read "I(B) 3"() -> (w332:cluster{dbl[], dbl[]}[])
                      n129 = Index Array(array=w332, index=0) -> (element=w331:cluster{dbl[], dbl[]})
                      n130 = Index Array(array=w332, index=1) -> (element=w333:cluster{dbl[], dbl[]})
                      n131 = local read "B array"() -> (w326:dbl[])
                      n132 = Index Array(array=w325, index=1) -> (element=w321:cluster{"B array":dbl[], dbl[]})
                      n133 = Unbundle(w331) -> (w329:dbl[], w330:dbl[])
                      n134 = Index Array(array=w325, index=0) -> (element=w322:cluster{"B array":dbl[], dbl[]})
                      n135 = Unbundle(w333) -> (w328:dbl[], w327:dbl[])
                      n136 = Unbundle(w321) -> ("B array"=w306:dbl[], w314:dbl[])
                      n137 = Unbundle(w322) -> ("B array"=w308:dbl[], w320:dbl[])
                      n138 = local read "Counter"() -> (w312:i8)
                      n139 = call <vilib>:"Interpolate 1D.vi"("xi"=w326, "X"=w328, "Y"=w327) -> ("yi"=w310:dbl[])  [unwired: 6 in, 2 out]
                      n140 = call <vilib>:"Interpolate 1D.vi"("xi"=w326, "X"=w329, "Y"=w330) -> ("yi"=w317:dbl[])  [unwired: 6 in, 2 out]
                      n141 = Decrement(x=w312) -> (x-1=w319:i8)
                      n142 = Decrement(x=w312) -> (x-1=w313:i8)
                      n143 = Multiply(x=w320, y=w319) -> (x*y=w318:dbl[])
                      n144 = Multiply(x=w314, y=w313) -> (x*y=w311:dbl[])
                      n145 = Add(x=w318, y=w317) -> (x+y=w316:dbl[])
                      n146 = Add(x=w310, y=w311) -> (x+y=w315:dbl[])
                      n147 = Divide(x=w316, y=w312) -> (x/y=w309:dbl[])
                      n148 = Divide(x=w315, y=w312) -> (x/y=w307:dbl[])
                      n149 = Bundle("B array"=w306, w307) -> (w304:cluster{"B array":dbl[], dbl[]})  [unwired: 1 in]
                      n150 = Bundle("B array"=w308, w309) -> (w305:cluster{"B array":dbl[], dbl[]})  [unwired: 1 in]
                      n151 = Build Array(w305, w304) -> (→"I(B) /Averaged/":cluster{"B array":dbl[], dbl[]}[])
                    }
                    frame #1 {
                      # "Save and Reset"
                      n152 = Build Array(w342, w338, w339, w337) -> (w336:dbl[][])
                      n153 = local read "output array"() -> (w341:dbl[][])
                      n154 = local write "Reset"(FALSE ("Save")) -> ()
                      n155 = Build Array (concatenate)(w341, w336) -> (→"output array":dbl[][])
                    }
                  }
                }
              }
            }
            frame "Return" {
            }
          }
        }
      }
      frame Error {
        # "Return true for any case which should stop the loop."
      }
    }
  }
  n156 = while {
    shift-right: [w373] -> w28
    shift-left: w4 -> [w374]
    shift-right: [w375] -> w35
    shift-left: w36 -> [w376]
    tunnel: w31 -> [w372]
    tunnel: w30 -> [w371]
    tunnel: w7 -> [w370]
    tunnel: [w364] -> _
    tunnel: w15 -> [w363]
    tunnel: w2 -> [w362]
    stop <- "stop" stop-if-true
    n157 = event shown="[7] \"Calibrate\": Value Change" {
      selector: _ -> [_ _ _ _ _ _ _ _ _ _ _ _ _]
      dyn-events: _ -> [_ _ _ _ _ _ _ _ _ _ _ _ _]
      timeout: 10 -> [_ _ _ _ _ _ _ _ _ _ _ _ _]
      tunnel: w376 -> [w386 w419 w429 w437 w448 w452 w477 _ w530 w537 w553 w563 w574]
      tunnel: [w385 w419 w429 w437 w448 w452 w477 _ w530 w537 w553 w563 w574] -> w375
      tunnel: w374 -> [w384 w418 w428 w438 w447 w456 w476 _ w531 w539 w557 w567 w576]
      tunnel: [w383 w418 w428 w438 w449 w456 w476 _ w531 w538 w556 w566 w575] -> w373
      tunnel: w372 -> [w382 _ _ _ _ _ _ _ _ _ _ _ _]
      tunnel: w371 -> [w381 _ _ _ _ _ _ _ _ _ _ _ _]
      tunnel: w370 -> [w380 _ _ _ _ _ _ _ _ _ _ _ _]
      tunnel: [w378 w417 w427 w436 w450 w453 w475 _ w529 w536 w554 w564 _] -> w364
      tunnel: w363 -> [w378 w417 w430 w436 w450 w453 w475 _ w529 w536 w554 w564 _]
      tunnel: w362 -> [_ _ _ _ _ _ _ _ _ w540 w555 w568 w573]
      event Timeout {
        n158 = event-data() -> ()  [unwired: 1 in, 3 out]
        n159 = case shown="True" "Measuring" {
          tunnel: w386 -> [w388 w407]
          tunnel: [w388 w406] -> w385
          tunnel: w384 -> [w387 _]
          tunnel: [w387 w405] -> w383
          tunnel: w382 -> [_ w398]
          tunnel: w381 -> [_ w397]
          tunnel: w380 -> [_ w392]
          frame False {
          }
          frame True {
            w395 = ":FETCh? " ("data")
            w399 = u32 1000 ("byte count")
            # "Generate the data here."
            n160 = case shown="No Error" w392 {
              selector: w392 -> [w409 w410]
              tunnel: [w409 w410] -> w391
              tunnel: [w408 _] -> w390
              frame No Error {
                n161 = Get Date/Time In Seconds() -> (seconds since 1Jan1904=w408:timestamp)
              }
              frame Error {
              }
            }
            n162 = VISA Write(VISA resource name=w398, write buffer=w395, error in (no error)=w391) -> (VISA resource name out=w404:refnum<visa-resource-name>, error out=w402:errorcluster)  [unwired: 1 out]
            n163 = VISA Write(VISA resource name=w397, write buffer=w395, error in (no error)=w402) -> (VISA resource name out=w403:refnum<visa-resource-name>, error out=w401:errorcluster)  [unwired: 1 out]
            n164 = VISA Read(VISA resource name=w404, byte count=w399, error in (no error)=w401) -> (read buffer=w393:string, error out=w400:errorcluster)  [unwired: 2 out]
            n165 = VISA Read(VISA resource name=w403, byte count=w399, error in (no error)=w400) -> (read buffer=w394:string, error out=w396:errorcluster)  [unwired: 2 out]
            n166 = Bundle("seconds since 1Jan1904"=w390, "read buffer"=w393, "read buffer"=w394) -> (w389:T5)  [unwired: 1 in]
            n167 = Enqueue Element(queue=w407, element=w389, error in (no error)=w396) -> (queue out=w406:refnum<queue>, error out=w405:errorcluster)  [unwired: 1 in, 1 out]
          }
        }
      }
      event "Max Field (T)": Value Change {
        n168 = event-data() -> ()  [unwired: 1 in, 6 out]
        n169 = Divide(x="Max Field (T)", y="dB (T)") -> (x/y=w414:dbl)
        n170 = Increment(x=w414) -> (x+1=w413:dbl)
        n171 = for {
          N: w413 -> [_]
          tunnel: "dB (T)" -> [w424]
          tunnel: [w421] -> w412 mode=indexing
          tunnel: "Min Field (T)" -> [w422]
          tunnel: [0.0] -> _ mode=indexing
          i -> [w426]
          n172 = Decrement(x=w426) -> (x-1=w425:i32)
          n173 = Multiply(x=w425, y=w424) -> (x*y=w423:dbl)
          n174 = Add(x=w423, y=w422) -> (x+y=w421:dbl)
        }
        "B array" <- w412
      }
      event "Sweep Rate (T/min)": Value Change {
        n175 = event-data() -> ("NewVal"=w434:dbl)  [unwired: 1 in, 5 out]
        n176 = Number To Fractional String(number=w434, precision (6)=i16 3) -> (F-format string=w432:string)  [unwired: 2 in]
        n177 = Concatenate Strings("T" ("format string"), w432) -> (w431:string)
        n178 = call "GPIB - BusCommand.vi"("Command"=w431, "Address"=w430) -> ("Address(thru)"=w427:T4)  [unwired: 1 out]
      }
      event "Field To Zero": Value Change {
        n179 = event-data() -> ()  [unwired: 1 in, 6 out]
        n180 = Two Button Dialog(message="Do you want to switch off the field?", 1:"No" ("F button name (\"Cancel\")"), 2:"Yes" ("T button name (\"OK\")")) -> (T button?=w442:bool)
        n181 = case shown="True" w442 {
          tunnel: w436 -> [_ w445]
          frame False {
          }
          frame True {
            n182 = local read "Sweep Rate (T/min)"() -> (w444:dbl)
            n183 = call "ips_switchHeaterOff.vi"("Instrument address"=w445, "Rate"=w444) -> ("B"=w443:dbl)
            n184 = local write "Actual Field (T)"(w443) -> ()
          }
        }
      }
      event "Go to Set": Value Change {
        n185 = event-data() -> ()  [unwired: 1 in, 6 out]
        n186 = call "Set_B.vi"("error in (no error)"=w447, "address string"="25", "Set Field (T)"="Set Field (T)") -> ("error out"=w449:errorcluster)  [unwired: 8 in]
      }
      event "Measure (Start/Pause)": Value Change {
        n187 = event-data() -> ("OldVal"=w454:bool, "NewVal"=w455:bool)  [unwired: 1 in, 4 out]
        n188 = local write "Measuring"(w455) -> ()
        n189 = case shown="True" w454 {
          frame False {
            n190 = local write "Temperature array"(dbl[] []) -> ()
          }
          frame True {
            # "Save data"
            n191 = case shown="False" "Temp/Magnetic Field" {
              tunnel: [w464 w473] -> w459
              frame False {
                n192 = local read "output array"() -> (w464:dbl[][])
              }
              frame True {
                n193 = local read "Magnetic Field (T)"() -> (w474:dbl[])
                n194 = local read "Measured Current (pA)"() -> (w472:dbl[])
                n195 = local read "Elapsed Time (s)"() -> (w469:dbl[])
                n196 = local read "Temperature array"() -> (w470:dbl[])
                n197 = call "Integrate_dPdt.vi"("Measured Current (pA)"=w472, "Sample area (mm^2)"="Sample area (mm^2)", "Temperature array"=w470, "Elapsed Time (s)"=w469, "dt (s)"="dt (s)") -> ("P(T)"=w468:cluster{"Temperature array":dbl[], dbl[]})  [unwired: 4 in, 2 out]
                "P(T)" <- w468
                n198 = Unbundle(w468) -> ("Temperature array"=w467:dbl[], w466:dbl[])
                n199 = Build Array(w470, w474, w472, w469, w467, w466) -> (w473:dbl[][])
              }
            }
            n200 = local read "Measurement File"() -> (w461:path)
            n201 = call-poly <vilib>:"Write Delimited Spreadsheet.vi"("file path (dialog if empty)"=w461, "format (%.3f)"="%.5g", "2D data"=w459, "append to file? (F)"=TRUE, "transpose? (F)"=TRUE) -> ()  [unwired: 9 in, 2 out]
          }
        }
      }
      event "Measure Noise": Value Change {
        n202 = event-data() -> ("NewVal"=w478:bool)  [unwired: 1 in, 5 out]
        n203 = case shown="True" w478 {
          frame False {
          }
          frame True {
            n204 = local read "Gain (V/A)"() -> (w483:dbl)
            n205 = call "Noise_measurement.vi"("Gain (V/A)"=w483, "Cycles"="Cycles", "Lower Cut-Off"="Cut-Off Frequency", "minimum value"="minimum value", "Filter On"="Filter On", "maximum value"="maximum value", "physical channels"="physical channels", "rate"="Rate", "samples per channel"="Samples per channel") -> ("Current (pA) Filtered"=→"Current (pA) Filtered":waveform(dbl), "PSD (pA/Hz^1/2) Peaks Removed"=→"PSD (pA/Hz^1/2) Peaks Removed":cluster{"f0":dbl, "df":dbl, "magnitude":dbl[]}, "Current (pA)"=→"Current (pA)":dbl[], "PSD (pA/Hz^1/2)"=→"PSD (pA/Hz^1/2)":cluster{"f0":dbl, "df":dbl, "magnitude":dbl[]})  [unwired: 3 in]
          }
        }
      }
      event "Calibrate": Value Change {
        n206 = event-data() -> ()  [unwired: 1 in, 6 out]
        n207 = case shown="True" "Calibrate" {
          frame False {
          }
          frame True {
            w495 = dbl[] []
            n208 = while {
              shift-right: [w528] -> w493
              shift-left: dbl[][] [] -> [w527]
              shift-right: [w511] -> _
              shift-left: w495 -> [w523]
              shift-right: [w520] -> _
              shift-left: w495 -> [w522]
              shift-right: [w510] -> _
              shift-left: w495 -> [w521]
              shift-right: [w502] -> _
              shift-left: 0.0 ("Set Field out") -> [w501]
              stop <- w524 stop-if-true
              n209 = call "Calibtarion.vi"("Dwell Time (ms)"="Dwell Time (ms)", "V array in (V)"=w523, "I array in (A)"=w521, "Collected array in"=w527, "B array in (T)"=w522, "Set Field (T)"=w501, "dB"="dB") -> ("Best Linear Fit"=w512:dbl[], "appended array"=→"appended array":dbl[][], "slope"=→"B/V (T/V)":dbl, "V array out (V)"=w511:dbl[], "Boolean"=w526:bool, "I array out (A)"=w510:dbl[], "intercept 2"=→"I0 (A)":dbl, "Collected array out"=w528:dbl[][], "intercept"=→"B0 (T)":dbl, "B array Out"=w520:dbl[], "slope 2"=→"V/I (Ohm)":dbl, "Best Linear Fit 2"=w517:dbl[], "Set Field out"=w502:dbl)
              n210 = Bundle("I array out (A)"=w510, "V array out (V)"=w511) -> (w519:T6)  [unwired: 1 in]
              n211 = Bundle("I array out (A)"=w510, "Best Linear Fit"=w512) -> (w513:T7)  [unwired: 1 in]
              n212 = Bundle("V array out (V)"=w511, "B array Out"=w520) -> (w515:T8)  [unwired: 1 in]
              n213 = Bundle("V array out (V)"=w511, "Best Linear Fit 2"=w517) -> (w516:T9)  [unwired: 1 in]
              n214 = Or(x=w526, y="stop 2") -> (x .or. y?=w524:bool)
              n215 = Build Array(w519, w513) -> (→"V_I":T10)
              n216 = Build Array(w515, w516) -> (→"B_V":T11)
            }
            n217 = flat-sequence {
              tunnel: w493 -> [w499]
              frame #0 {
                n218 = Two Button Dialog(message="Do you want to save calibration file?") -> (T button?=w498:bool)  [unwired: 2 in]
                n219 = case shown="True" w498 {
                  tunnel: w499 -> [_ w500]
                  frame False {
                  }
                  frame True {
                    n220 = call-poly <vilib>:"Write Delimited Spreadsheet.vi"("2D data"=w500) -> ()  [unwired: 13 in, 2 out]
                  }
                }
              }
            }
          }
        }
      }
      event "New Measurement File": Value Change {
        n221 = event-data() -> ()  [unwired: 1 in, 6 out]
        n222 = Open/Create/Replace File(prompt="Please select measurement file\n", operation (0:open)=T3."replace or create with confirmation") -> (refnum out=w532:refnum<file>)  [unwired: 4 in, 2 out]
        n223 = local write "refnum out"(w532) -> ()
        n224 = Refnum to Path(1:w532) -> (0:w533:path)
        n225 = call "File_header_diag.vi"("Byte Stream File in"=w532) -> ()  [unwired: 11 in]
        n226 = local write "Measurement File"(w533) -> ()
      }
      event "Heater On/Off": Value Change {
        n227 = event-data() -> ()  [unwired: 1 in, 6 out]
        n228 = case shown="True" "Heater On/Off" {
          tunnel: w540 -> [w545 w551]
          tunnel: w539 -> [w543 w552]
          tunnel: [w542 w550] -> w538
          frame False {
            n229 = VISA Write(VISA resource name=w545, write buffer="RANGE,1,0", error in (no error)=w543) -> (error out=w542:errorcluster)  [unwired: 2 out]
          }
          frame True {
            n230 = Number To Decimal String(number="Heater Range") -> (decimal integer string=w548:string)  [unwired: 1 in]
            n231 = Concatenate Strings("RANGE,1," ("write buffer"), w548) -> (w546:string)
            n232 = VISA Write(VISA resource name=w551, write buffer=w546, error in (no error)=w552) -> (error out=w550:errorcluster)  [unwired: 2 out]
          }
        }
      }
      event "Set temperature (K)": Value Change {
        n233 = event-data() -> ()  [unwired: 1 in, 6 out]
        n234 = local read "Set temperature (K)"() -> (w558:dbl)
        n235 = Number To Fractional String(number=w558, precision (6)=i16 3) -> (F-format string=w561:string)  [unwired: 2 in]
        n236 = Concatenate Strings("SETP 1," ("write buffer"), w561) -> (w559:string)
        n237 = VISA Write(VISA resource name=w555, write buffer=w559, error in (no error)=w557) -> (error out=w556:errorcluster)  [unwired: 2 out]
      }
      event "Temp Ramping Rate (K/min)": Value Change {
        n238 = event-data() -> ()  [unwired: 1 in, 6 out]
        n239 = local read "Temp Ramping Rate (K/min)"() -> (w565:dbl)
        n240 = Number To Fractional String(number=w565, precision (6)=i16 1) -> (F-format string=w571:string)  [unwired: 2 in]
        n241 = Concatenate Strings("RAMP 1,1," ("string"), w571) -> (w570:string)
        n242 = VISA Write(VISA resource name=w568, write buffer=w570, error in (no error)=w567) -> (error out=w566:errorcluster)  [unwired: 2 out]
      }
      event "Heater Range": Value Change {
        n243 = event-data() -> ()  [unwired: 1 in, 6 out]
        n244 = local read "Heater On/Off"() -> (w577:bool)
        n245 = case shown="False" w577 {
          tunnel: w576 -> [w578 w583]
          tunnel: [w578 w582] -> w575
          tunnel: w573 -> [_ w581]
          frame False {
          }
          frame True {
            n246 = local read "Heater Range"() -> (w579:enum16{"Off", "Low", "Medium", "High"})
            n247 = Number To Decimal String(number=w579) -> (decimal integer string=w585:string)  [unwired: 1 in]
            n248 = Concatenate Strings("RANGE,1," ("write buffer"), w585) -> (w584:string)
            n249 = VISA Write(VISA resource name=w581, write buffer=w584, error in (no error)=w583) -> (error out=w582:errorcluster)  [unwired: 2 out]
          }
        }
      }
    }
    n250 = Reciprocal(x="Sampling rate (Hz)") -> (1/x=w368:dbl)
    n251 = Multiply(x=w368, y=1000.0) -> (x*y=w366:dbl)
    n252 = Wait Until Next ms Multiple(millisecond multiple=w366) -> ()  [unwired: 1 out]
  }
  n253 = local read "Lake Shore"() -> (w5:refnum<visa-resource-name>)
  n254 = local read "IV converter"() -> (w26:refnum<visa-resource-name>)
  n255 = local read "Magnetic Field"() -> (w25:refnum<visa-resource-name>)
  n256 = VISA Close(VISA resource name=w26, error in (no error)=w28) -> (error out=w29:errorcluster)
  n257 = VISA Close(VISA resource name=w25, error in (no error)=w29) -> (error out=w27:errorcluster)
  n258 = Release Queue(queue=w35, error in (no error)=w27) -> (error out=w21:errorcluster)  [unwired: 1 in, 2 out]
  n259 = Merge Errors(w21, w20) -> (w22:errorcluster)
  n260 = VISA Close(VISA resource name=w5, error in (no error)=w22) -> (error out=w19:errorcluster)
  n261 = local read "refnum out"() -> (w17:refnum<file>)
  n262 = Close File(refnum=w17, error in=w19) -> (error out=w18:errorcluster)  [unwired: 1 out]
  n263 = call <vilib>:"Simple Error Handler.vi"("error in (no error)"=w18) -> ()  [unwired: 4 in, 5 out]
